vi "car3udpmsgtest02.vi"() -> ()   [LabVIEW 2020]
panel:
  in  "let-it-fail":bool
  in  "stop":bool
  in  "msg_type":u8
  in  "data (bytes string)":string="SB"
  in  "receiver_port":u16=16164
  in  "receiver_IPv4":string="192.168.1.64"
  out "sender_port":u16=16101
  out "sender_IPv4":string="192.168.1.1"
  out "message_bytes":string
  # "A test to check the state manager on the cRIO"
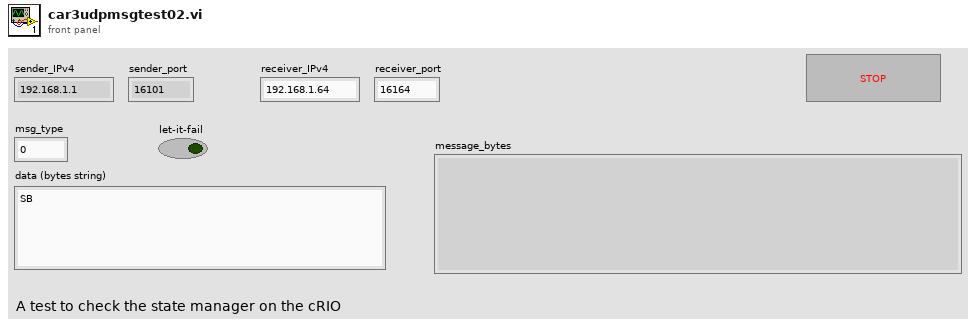
[diagram p1: front panel]
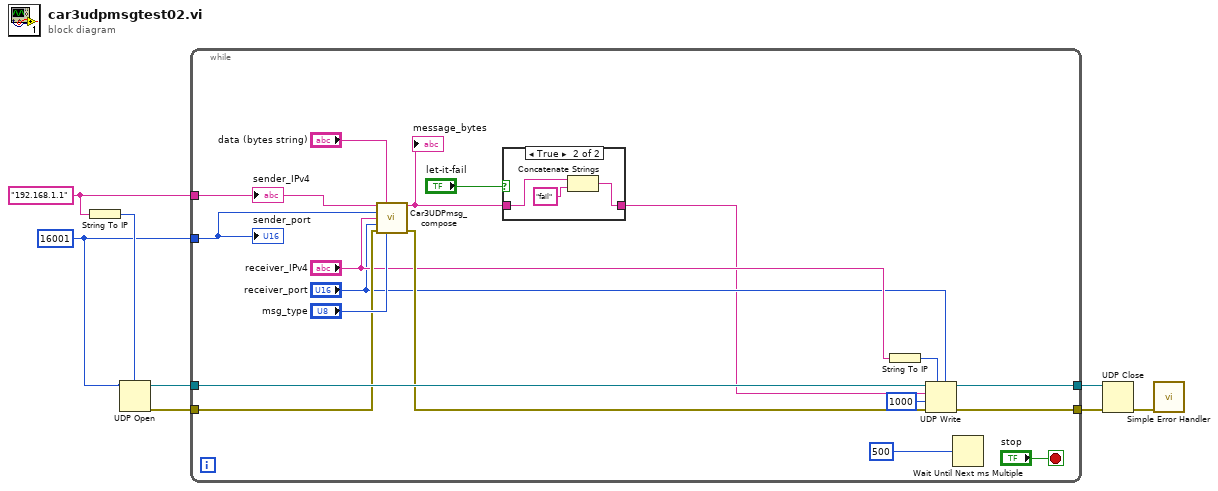
[diagram p0: block diagram]
diagram:
  w7 = "192.168.1.1" ("sender_IPv4")
  w1 = u16 16001 ("sender_port")
  n1 = String To IP(1:w7) -> (0:w2:u32)
  n2 = UDP Open(7:w2, 11:w1) -> (port=w4:refnum<k16>, 0:w3:errorcluster)  [unwired: 3 in, 1 out]
  n3 = while {
    tunnel: w7 -> [w20]
    tunnel: w1 -> [w19]
    tunnel: w4 -> [w18]
    tunnel: [w17] -> w6
    tunnel: w3 -> [w16]
    tunnel: [w10] -> w5
    stop <- "stop" stop-if-true
    n4 = call "Car3UDPmsg_compose.vi"("sender_IPv4"=w20, "data (bytes string)"="data (bytes string)", "sender_port"=w19, "receiver_IPv4"="receiver_IPv4", "receiver_port"="receiver_port", "error in (no error)"=w16, "msg_type"="msg_type") -> ("message_bytes"=w21:string, "error out"=w15:errorcluster)  [unwired: 6 in, 1 out]
    "message_bytes" <- w21
    n5 = case shown="True" "let-it-fail" {
      tunnel: w21 -> [w27 w29]
      tunnel: [w27 w30] -> w11
      frame False {
      }
      frame True {
        n6 = Concatenate Strings(w29, "fail" ("string")) -> (w30:string)
      }
    }
    n7 = String To IP(1:"receiver_IPv4") -> (0:w14:u32)
    n8 = UDP Write(address=w14, port or service name="receiver_port", connection ID=w18, data in=w11, 8:w15, 9:1000 ("timeout ms (25000)")) -> (error out=w10:errorcluster, 3:w17:refnum<k16>)
    n9 = Wait Until Next ms Multiple(millisecond multiple=u32 500) -> ()  [unwired: 1 out]
    "sender_IPv4" <- w20
    "sender_port" <- w19
  }
  n10 = UDP Close(connection ID=w6, 8:w5) -> (error out=w8:errorcluster)  [unwired: 1 out]
  n11 = call <vilib>:"Simple Error Handler.vi"("error in (no error)"=w8) -> ()  [unwired: 4 in, 5 out]
